vi "event_quit.vi"(8 "error in":errorcluster, 9 "reference cluster in":T1) -> (0 "error out":errorcluster)   [LabVIEW 2016]
uses:
  Type Definitions/reference_cluster.ctl
  Type Definitions/vars_settings.ctl
  Type Definitions/stim_type.ctl
  Type Definitions/backlight_type.ctl
  Type Definitions/vars_runtime.ctl
  Type Definitions/data.ctl
  Type Definitions/notifier_elements_GUI.ctl
  Type Definitions/notifier_elements_DAQ.ctl
  Type Definitions/notifier_elements_write.ctl
  Type Definitions/control_references.ctl
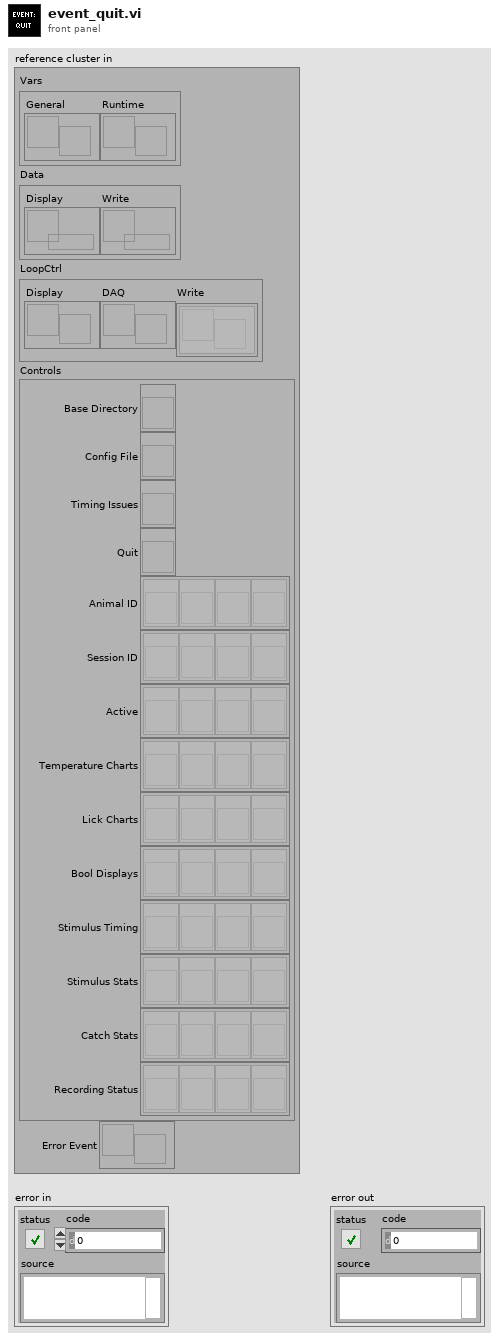
[diagram p1: front panel]
types:
  T1 = typedef "reference_cluster.ctl" = cluster{"Vars":cluster{"General":refnum<notifier>, "Runtime":refnum<notifier>}, "Data":cluster{"Display":refnum<queue>, "Write":refnum<queue>}, "LoopCtrl":cluster{"Display":refnum<notifier>, "DAQ":refnum<notifier>, "Write":refnum<notifier>[]}, "Controls":T2, "Error Event":refnum<user-event>}
  T2 = typedef "control_references.ctl" = cluster{"Base Directory":refnum<vi>, "Config File":refnum<vi>, "Timing Issues":refnum<vi>, "Quit":refnum<vi>, "Animal ID":refnum<vi>[], "Session ID":refnum<vi>[], "Active":refnum<vi>[], "Temperature Charts":refnum<vi>[], "Lick Charts":refnum<vi>[], "Bool Displays":refnum<vi>[], "Stimulus Timing":refnum<vi>[], "Stimulus Stats":refnum<vi>[], "Catch Stats":refnum<vi>[], "Recording Status":refnum<vi>[]}
  T3 = typedef "notifier_elements_write.ctl" = enum16{"Initialize", "Pause", "Write Data", "Close Files", "Quit"}
  T4 = typedef "notifier_elements_GUI.ctl" = enum16{"Initialize GUI", "Pause", "Live Update", "Stat Update", "Quit"}
  T5 = typedef "notifier_elements_DAQ.ctl" = enum16{"DAQ - Initialize", "DAQ - Pause", "DAQ - Run", "DAQ - Quit"}
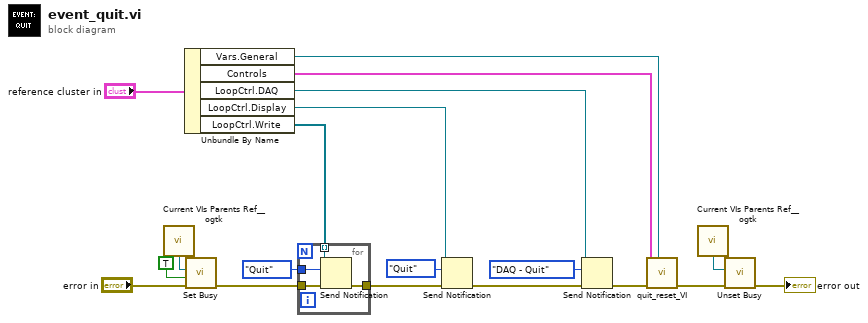
[diagram p0: block diagram]
diagram:
  n1 = call <userlib>:"Current VIs Parents Ref__ogtk.vi"() -> ("Calling VI's Reference"=w2:refnum<vi>)  [unwired: 2 in]
  n2 = Unbundle By Name("reference cluster in") -> ("Vars.General"=w19:refnum<notifier>, "Controls"=w17:T2, "LoopCtrl.DAQ"=w13:refnum<notifier>, "LoopCtrl.Display"=w12:refnum<notifier>, "LoopCtrl.Write"=w16:refnum<notifier>[])
  n3 = call <vilib>:"Set Busy.vi"("error in (no error)"="error in", "disable click? (T)"=TRUE, "VI reference (current VI)"=w2) -> ("error out"=w5:errorcluster)  [unwired: 7 in, 1 out]
  n4 = for {
    tunnel: [w23] -> w15
    tunnel: w16 -> [w22] mode=indexing
    tunnel: notifier_elements_write."Quit" ("notification") -> [w21]
    tunnel: w5 -> [w20]
    n5 = Send Notification(notification=w21, notifier=w22, error in (no error)=w20) -> (error out=w23:errorcluster)  [unwired: 1 out]
  }
  n6 = Send Notification(notification=notifier_elements_GUI."Quit", notifier=w12, error in (no error)=w15) -> (error out=w8:errorcluster)  [unwired: 1 out]
  n7 = Send Notification(notification=notifier_elements_DAQ."DAQ - Quit", notifier=w13, error in (no error)=w8) -> (error out=w18:errorcluster)  [unwired: 1 out]
  n8 = call "quit_reset_VI.vi"("Controls"=w17, "error in"=w18, "notifier"=w19) -> ("error out"=w3:errorcluster)  [unwired: 7 in]
  n9 = call <userlib>:"Current VIs Parents Ref__ogtk.vi"() -> ("Calling VI's Reference"=w6:refnum<vi>)  [unwired: 2 in]
  n10 = call <vilib>:"Unset Busy.vi"("error in (no error)"=w3, "VI reference (current VI)"=w6) -> ("error out"=→"error out":errorcluster)  [unwired: 9 in]
